vi "Function Generator.vi"(0 "Setpoint Source":T1(radio), 5 "Manual \nSetpoint in":sgl, 7 "Signal\nParameters":T2) -> (4 "Setpoint out":sgl)   [LabVIEW 2014]
uses:
  <vilib>/measure/NI_MABase.lvlib
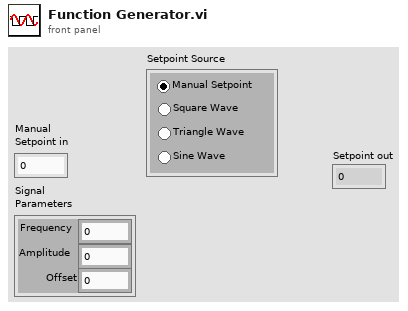
[diagram p1: front panel]
types:
  T1 = enum32{"Manual Setpoint", "Square Wave", "Triangle Wave", "Sine Wave"}
  T2 = cluster{"Frequency":sgl, "Amplitude":sgl, "Offset":sgl}
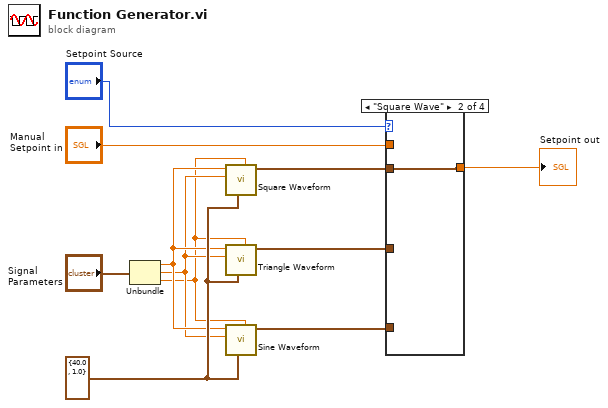
[diagram p0: block diagram]
diagram:
  w6 = cluster{"Fs":dbl, "#s":dbl} {"Fs"=40.0, "#s"=1.0} ("sampling info")
  n1 = Unbundle("Signal\nParameters") -> ("Frequency"=w5:sgl, "Amplitude"=w4:sgl, "Offset"=w2:sgl)
  n2 = call <vilib>:"Square Waveform.vi"("offset"=w2, "sampling info"=w6, "amplitude"=w4, "frequency"=w5) -> ("signal out"=w9:waveform(dbl))  [unwired: 6 in, 1 out]
  n3 = call <vilib>:"Triangle Waveform.vi"("offset"=w2, "sampling info"=w6, "amplitude"=w4, "frequency"=w5) -> ("signal out"=w10:waveform(dbl))  [unwired: 6 in, 1 out]
  n4 = call <vilib>:"Sine Waveform.vi"("offset"=w2, "sampling info"=w6, "amplitude"=w4, "frequency"=w5) -> ("signal out"=w11:waveform(dbl))  [unwired: 6 in, 1 out]
  n5 = case shown="\"Square Wave\"" "Setpoint Source" {
    tunnel: "Manual \nSetpoint in" -> [w12 _ _ _]
    tunnel: [w12 w13 w14 w15] -> w8
    tunnel: w9 -> [_ w13 _ _]
    tunnel: w10 -> [_ _ w14 _]
    tunnel: w11 -> [_ _ _ w15]
    frame "Manual Setpoint", Default {
    }
    frame "Square Wave" {
    }
    frame "Triangle Wave" {
    }
    frame "Sine Wave" {
    }
  }
  "Setpoint out" <- w8
